vi "test.vi"() -> ()   [LabVIEW 2020]
panel:
  out "num_passed":i32
  out "num_tested":i32
  out "error type":enum16{"fatal", "non-fatal", "warning"}(ring)
  in  "VIs without test coverage":i32(listbox)
  out "error out":errorcluster
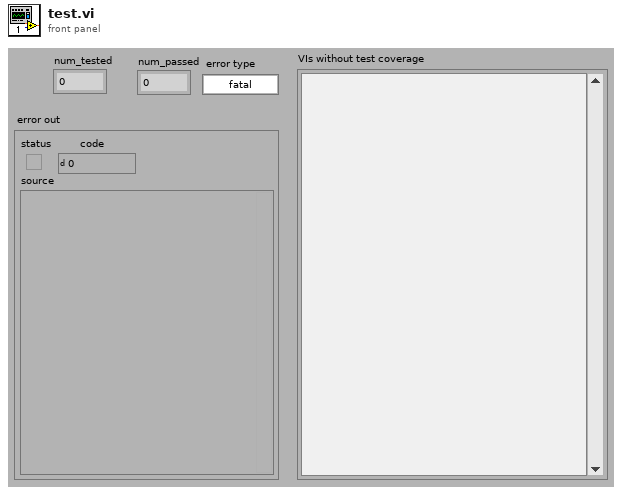
[diagram p1: front panel]
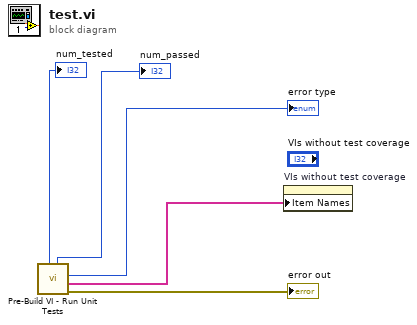
[diagram p0: block diagram]
diagram:
  n1 = call "Pre-Build VI - Run Unit Tests.vi"() -> ("error out"=→"error out":errorcluster, "VIs without test coverage"=w4:string[], "error type"=→"error type":enum16{"fatal", "non-fatal", "warning"}, "num_passed"=→"num_passed":i32, "num_tested"=→"num_tested":i32)  [unwired: 7 in]
  n2 = property on="VIs without test coverage" class="LstBox (strict)"("Item Names"=w4) -> ()  [unwired: 2 in, 2 out]
